vi "Merge Builds.vi"(8 "error in":errorcluster, 11 "Destination Path":path) -> (0 "error out":errorcluster)   [LabVIEW 2013]
doc: "This VI will look for builds of the same version number and copies the other builds' EXE files to this build. This VI should be called only from the main main build with all drivers or it may do some crazy stuff."
uses:
  <vilib>/regexp/Match Regular Expression.xnode
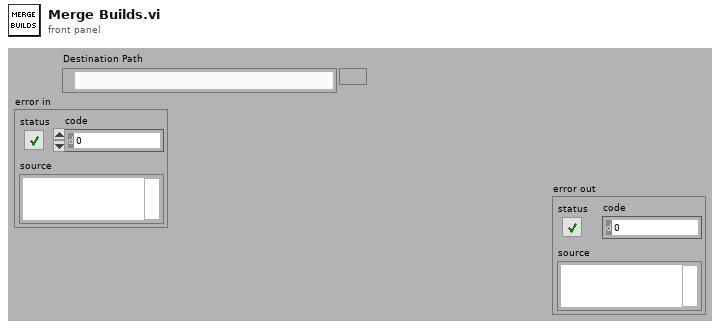
[diagram p1: front panel]
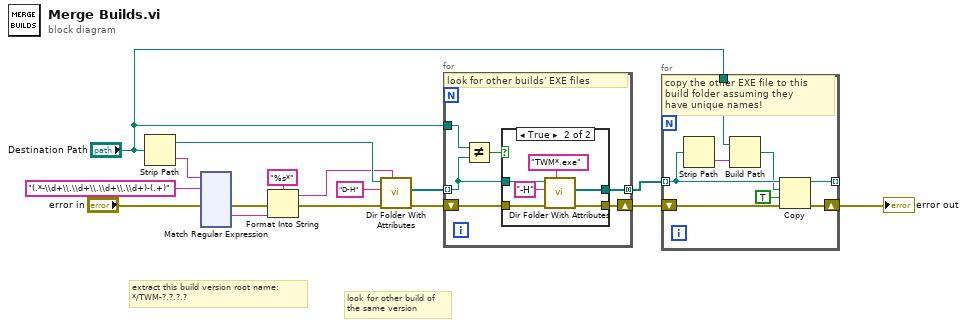
[diagram p0: block diagram]
diagram:
  # "look for other build of\nthe same version"
  # "extract this build version root name:\n*/TWM-?.?.?.?"
  n1 = Strip Path(path="Destination Path") -> (stripped path=w8:path, name=w16:string)
  n2 = xnode "Match Regular Expression"("input string"=w16, "regular expression"="(.*-\\d+\\.\\d+\\.\\d+\\.\\d+)-(.+)", "error in"="error in") -> ("error out"=w14:errorcluster, "submatch 1"=w10:string)  [unwired: 3 in, 5 out]
  n3 = Format Into String(format string="%s*", error in=w14, w10) -> (resulting string=w7:string, error out=w13:errorcluster)  [unwired: 1 in]
  n4 = call "Dir Folder With Attributes.vi"("wildcard serach key (*)"=w7, "error in (no error)"=w13, "\"DIR /A:?\" attribute(s) (default: -H)"="D-H" ("\"DIR /A:?\" attribute(s) (default: -H)"), "folder"=w8) -> ("error out"=w6:errorcluster, "file/folder paths"=w9:path[])  [unwired: 5 in, 1 out]
  n5 = for {
    tunnel: "Destination Path" -> [w22]
    tunnel: w9 -> [w20] mode=indexing
    shift-right: [w19] -> w4
    shift-left: w6 -> [w21]
    tunnel: [w18] -> w2 mode=concatenating
    # "look for other builds' EXE files"
    n6 = Not Equal?(x=w22, y=w20) -> (x != y?=w17:bool)
    n7 = case shown="True" w17 {
      tunnel: w21 -> [w23 w29]
      tunnel: w20 -> [_ w28]
      tunnel: [w23 w27] -> w19
      tunnel: [_ w24] -> w18
      frame False {
      }
      frame True {
        n8 = call "Dir Folder With Attributes.vi"("wildcard serach key (*)"="TWM*.exe", "error in (no error)"=w29, "\"DIR /A:?\" attribute(s) (default: -H)"="-H" ("\"DIR /A:?\" attribute(s) (default: -H)"), "folder"=w28) -> ("error out"=w27:errorcluster, "file/folder paths"=w24:path[])  [unwired: 5 in, 1 out]
      }
    }
  }
  n9 = for {
    shift-right: [w31] -> w3
    shift-left: w4 -> [w37]
    tunnel: w2 -> [w34] mode=indexing
    tunnel: "Destination Path" -> [w35]
    tunnel: [w30] -> _ mode=indexing
    # "copy the other EXE file to this\nbuild folder assuming they\nhave unique names!"
    n10 = Strip Path(path=w34) -> (name=w36:string)  [unwired: 1 out]
    n11 = Build Path(base path=w35, name or relative path=w36) -> (appended path=w33:path)
    n12 = Copy(8:w37, 9:TRUE ("overwrite (F)"), 10:w33, 11:w34) -> (0:w31:errorcluster, 3:w30:path)  [unwired: 1 in, 1 out]
  }
  "error out" <- w3
